vi "Lab2_Exercise2_Li_Lim.vi"() -> ()   [LabVIEW 2016]
panel:
  out "Meter":dbl(knob) scale=0.0..10.0
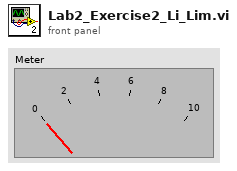
[diagram p1: front panel]
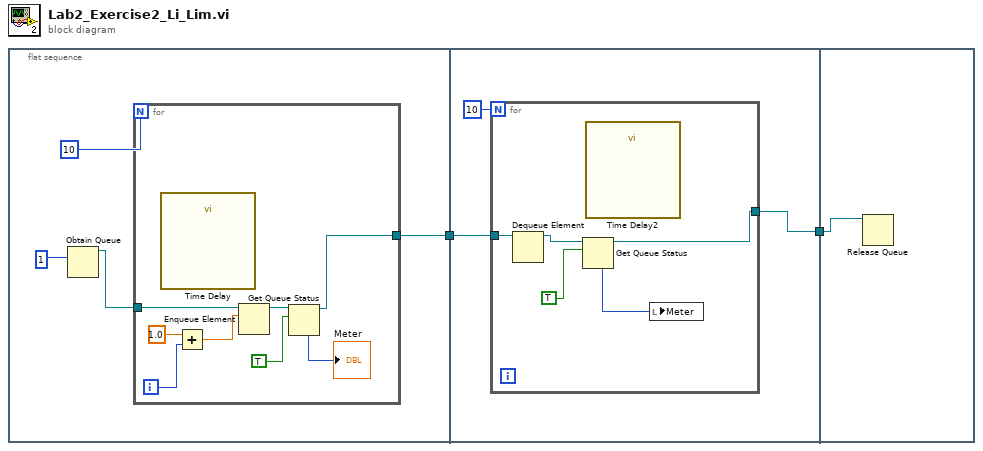
[diagram p0: block diagram]
diagram:
  n1 = flat-sequence {
    tunnel: [w3] -> w2
    tunnel: w2 -> [w17]
    tunnel: [w15] -> w1
    tunnel: w1 -> [w23]
    frame #0 {
      n2 = Obtain Queue(element data type=1) -> (queue out=w4:refnum<queue>)  [unwired: 4 in, 2 out]
      n3 = for {
        N: 10 -> [_]
        tunnel: w4 -> [w11]
        tunnel: [w7] -> w3
        i -> [w13]
        n4 = call "Time Delay"() -> ()  [unwired: 11 in, 1 out]
        n5 = Add(x=1.0, y=w13) -> (x+y=w12:dbl)
        n6 = Enqueue Element(queue=w11, element=w12) -> (queue out=w10:refnum<queue>)  [unwired: 2 in, 2 out]
        n7 = Get Queue Status(queue=w10, return elements? (F)=TRUE) -> (queue out=w7:refnum<queue>, # elements in queue=→"Meter":i32)  [unwired: 1 in, 6 out]
      }
    }
    frame #1 {
      n8 = for {
        N: 10 -> [_]
        tunnel: w17 -> [w22]
        tunnel: [w19] -> w15
        n9 = Dequeue Element(queue=w22) -> (queue out=w21:refnum<queue>)  [unwired: 2 in, 3 out]
        n10 = Get Queue Status(queue=w21, return elements? (F)=TRUE) -> (queue out=w19:refnum<queue>, # elements in queue=w18:i32)  [unwired: 1 in, 6 out]
        n11 = call "Time Delay2"() -> ()  [unwired: 11 in, 1 out]
        n12 = local write "Meter"(w18) -> ()
      }
    }
    frame #2 {
      n13 = Release Queue(queue=w23) -> ()  [unwired: 2 in, 3 out]
    }
  }
